vi "VSS Tangent.vi"(4 "Passe":bool, 6 "Cone de chute":dbl=0.55 format="%#_13g", 7 "IA State Input in":T1, 8 "distance between ball and robot":dbl=250.0 format="%#_13g", 9 "Ball":dbl[](array[numeric])=[-1986.6092529296875, -3009.6396484375], 10 "Target":dbl[](array[numeric]), 11 "R":dbl[](array[numeric])=[-2840.578369140625, -1536.7857666015625, -1.0371381044387817]) -> (1 "Destination":dbl[](array[numeric]))   [LabVIEW 2018]
uses:
  Core/AI Input.ctl
  Core/AI Robot.ctl
  Intel/Functions Enum.ctl
  Intel/AttackerStates.ctl
  Path Planning/RRT/PathDests.ctl
  Path Planning/RRT/PathDest.ctl
  Core/AI Ball.ctl
  Core/Field Size.ctl
  Core/AI Judge.ctl
  Intel/Command Enum.ctl
  Util/Events/Events.ctl
  <vilib>/Analysis/coordinate.llb/2D Cartesian Coordinate Rotation (Scalar).vi
  <vilib>/Analysis/NI_AALPro.lvlib
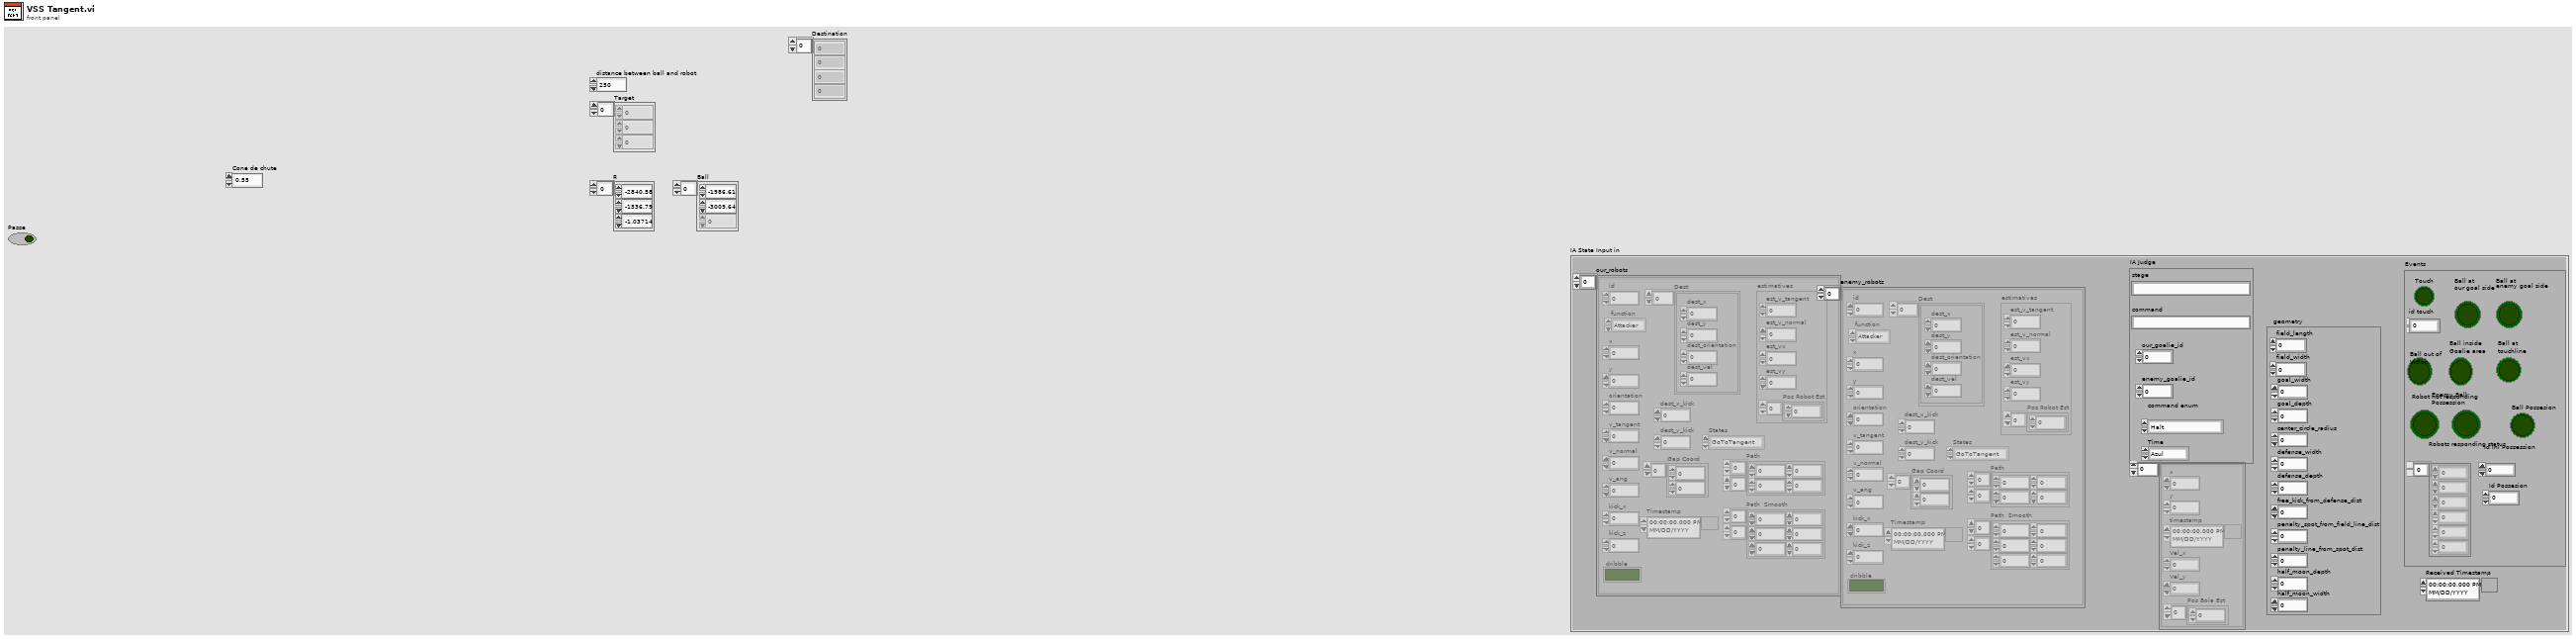
[diagram p1: front panel]
types:
  T1 = typedef "AI Input.ctl" = cluster{"our_robots":T2[], "enemy_robots":T2[], "balls":T7[], "geometry":T8, "IA Judge":T9, "Received Timestamp":timestamp, "Events":T11}
  T2 = typedef "AI Robot.ctl" = cluster{"id":u32, "function":T3, "x":dbl, "y":dbl, "orientation":dbl, "v_tangent":dbl, "v_normal":dbl, "v_ang":dbl, "kick_x":dbl, "kick_z":dbl, "dribble":bool, "Timestamp":timestamp, "estimatives":cluster{"est_v_tangent":dbl, "est_v_normal":dbl, "est_vx":dbl, "est_vy":dbl, "Pos Robot Est":dbl[]}, "dest_x_kick":dbl, "dest_y_kick":dbl, "Gap Coord":dbl[], "States":T4, "Path ":dbl[][], "Path  Smooth":dbl[][], "Dest":T5}
  T3 = typedef "Functions Enum.ctl" = enum16{"Attacker", "Goalie", "Defender", "Striker", "Goto 0", "Dummy", "Kicker", "ZigZag"}
  T4 = typedef "AttackerStates.ctl" = enum16{"Pass", "GoToTangent", "BallGetting", "GoToKick", "Rotate anti-clockwise", "Rotate Clockwise", ""}
  T5 = typedef "PathDests.ctl" = T6[]
  T6 = typedef "PathDest.ctl" = cluster{"dest_x":dbl, "dest_y":dbl, "dest_orientation":dbl, "dest_vel":dbl}
  T7 = typedef "AI Ball.ctl" = cluster{"x":dbl, "y":dbl, "timestamp":timestamp, "Vel_x":dbl, "Vel_y":dbl, "Pos Bola Est":dbl[]}
  T8 = typedef "Field Size.ctl" = cluster{"field_length":u32, "field_width":u32, "goal_width":u32, "goal_depth":u32, "center_circle_radius":u32, "defense_width":u32, "defense_depth":u32, "free_kick_from_defense_dist":u32, "penalty_spot_from_field_line_dist":u32, "penalty_line_from_spot_dist":u32, "half_moon_depth":u32, "half_moon_width":u32}
  T9 = typedef "AI Judge.ctl" = cluster{"stage":string, "command":string, "our_goalie_id":dbl, "enemy_goalie_id":dbl, "command enum":T10, "Time":enum16{"Azul", "Amarelo"}}
  T10 = typedef "Command Enum.ctl" = enum16{"Halt", "Stop", "Force Start", "PKA Normal Start", "Prepare Kickoff Ally", "PKE Normal Start", "Prepare Kickoff Enemy", "Prepare Penalty Ally", "PPA Normal Start", "Prepare Penalty Enemy", "PPE Normal Start", "Ball Placement Enemy Up", "Ball Placement Enemy Down", "Ball Placement Ally Up", "Ball Placement Ally Mid", "Ball Placement Ally Down", "Indirect Free Enemy", "Indirect Free Ally", "Timeout Enemy", "Timeout Ally", "Goal Enemy", "Goal Ally", "Normal Half Time", "Extra Time Break", "Extra Half Time", "None", "Post Game"}
  T11 = typedef "Events.ctl" = cluster{"Touch":bool, "id touch":dbl, "Ball out of \nVision":bool, "Ball inside \nGoalie area":bool, "Robot not responding":bool, "Robots responding status":dbl[], "Enemy Ball \nPossession":bool, "Id ini Possession":dbl, "Ball Possesion":bool, "Id Possesion":dbl, "Ball at\nour goal side":bool, "Ball at\ntouchline":bool, "Ball at\nenemy goal side":bool}
  T12 = enum16{"Frente", "Fundo", "Cima", "Baixo", "None"}
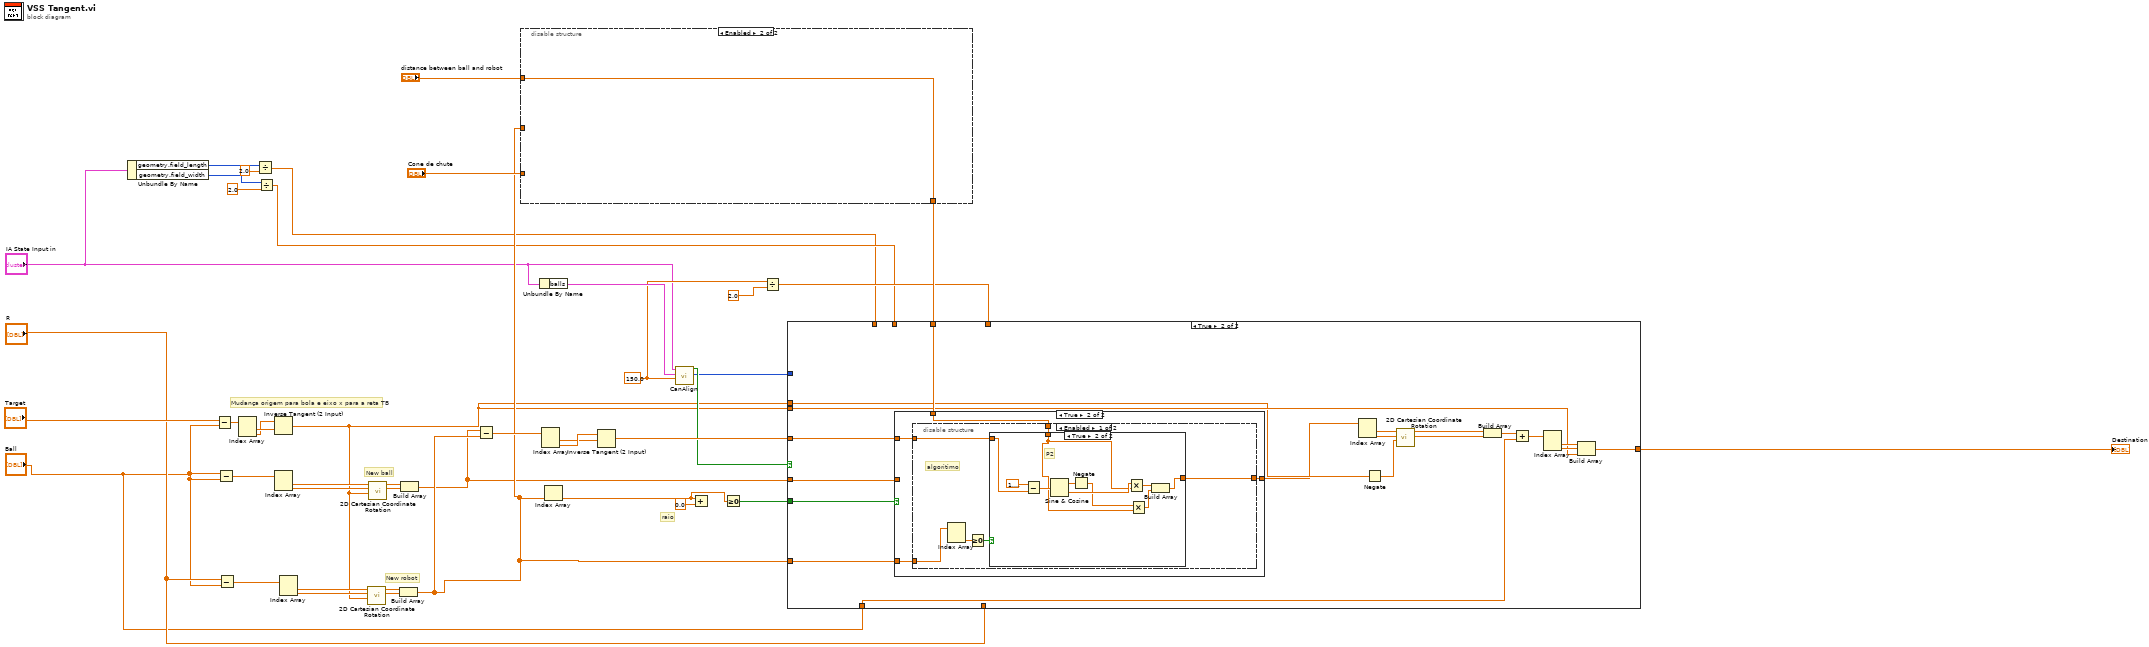
[diagram p0: block diagram]
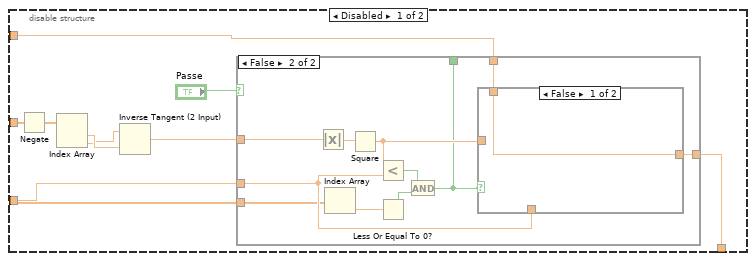
[diagram p2: hidden frame]
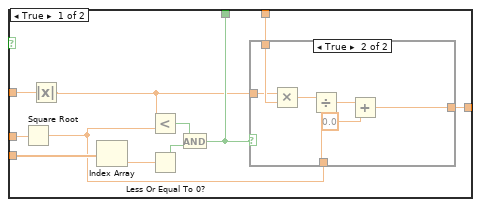
[diagram p3: hidden frame]
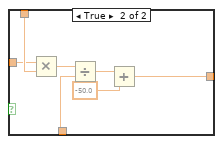
[diagram p5: hidden frame]
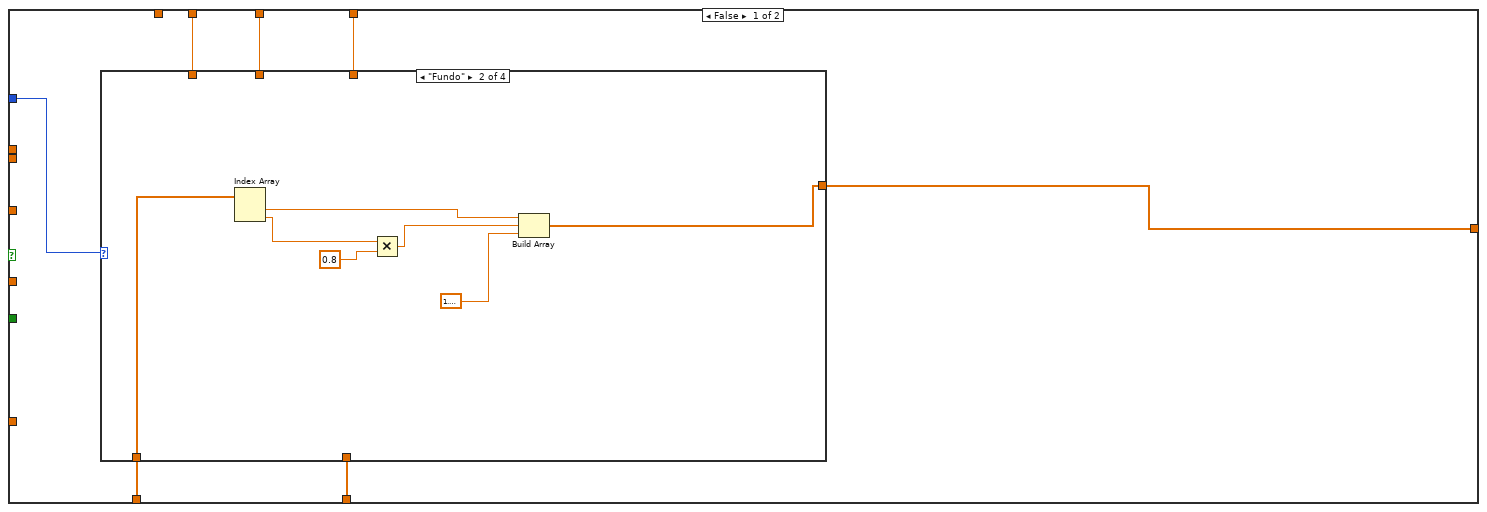
[diagram p6: hidden frame]
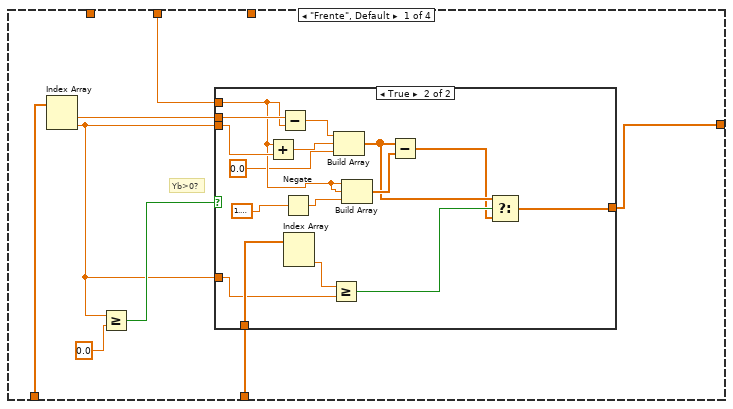
[diagram p7: hidden frame]
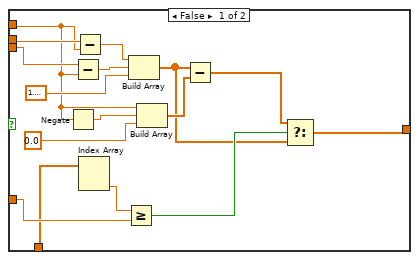
[diagram p8: hidden frame]
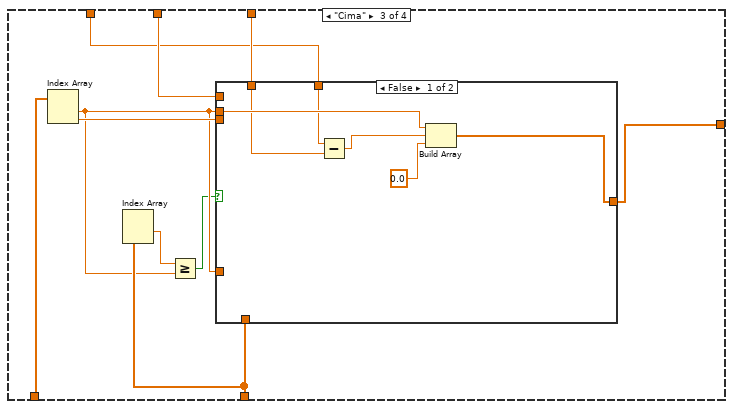
[diagram p9: hidden frame]
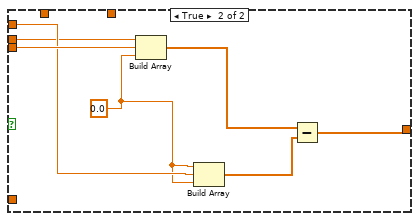
[diagram p10: hidden frame]
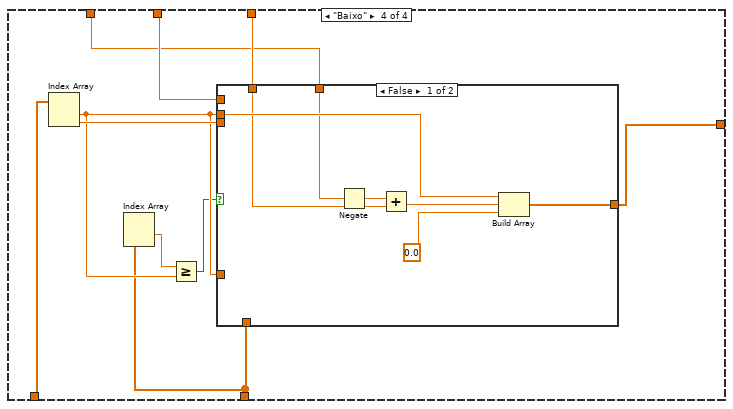
[diagram p11: hidden frame]
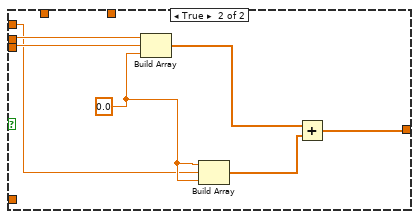
[diagram p12: hidden frame]
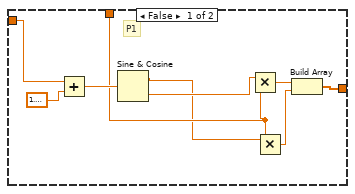
[diagram p14: hidden frame]
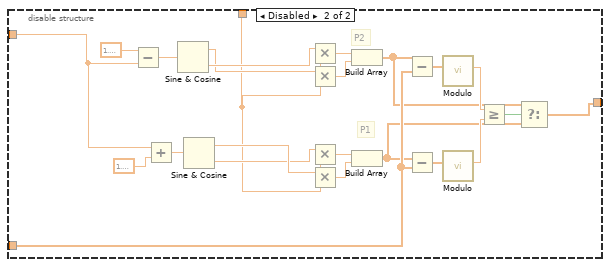
[diagram p15: hidden frame]
diagram:
  w12 = 150.0 ("Distância padrão\n de tolerância.")
  # "raio"
  # "New ball"
  # "New robot"
  # "Mudança origem para bola e eixo x para a reta TB"
  n1 = Unbundle By Name("IA State Input in") -> ("geometry.field_length"=w7:u32, "geometry.field_width"=w6:u32)
  n2 = Subtract(x="Target", y="Ball") -> (x-y=w37:dbl[])
  n3 = Subtract(x="Ball", y="Ball") -> (x-y=w41:dbl[])
  n4 = Subtract(x="R", y="Ball") -> (x-y=w38:dbl[])
  n5 = Index Array(array=w37) -> (element #1=w36:dbl, element #2=w35:dbl)  [unwired: 2 in]
  n6 = Divide(x=w7, y=2.0) -> (x/y=w4:dbl)
  n7 = Divide(x=w6, y=2.0) -> (x/y=w5:dbl)
  n8 = Inverse Tangent (2 Input)(1:w36, 2:w35) -> (0:w2:dbl)
  n9 = Index Array(array=w41) -> (element #1=w43:dbl, element #2=w42:dbl)  [unwired: 2 in]
  n10 = Index Array(array=w38) -> (element #1=w40:dbl, element #2=w39:dbl)  [unwired: 2 in]
  n11 = call-poly <vilib>:"2D Cartesian Coordinate Rotation.vi"("theta"=w2, "y"=w39, "x"=w40) -> ("y out"=w31:dbl, "x out"=w32:dbl)  [unwired: 6 in, 1 out]
  n12 = call-poly <vilib>:"2D Cartesian Coordinate Rotation.vi"("theta"=w2, "y"=w42, "x"=w43) -> ("y out"=w33:dbl, "x out"=w34:dbl)  [unwired: 6 in, 1 out]
  n13 = Build Array(w32, w31) -> (w23:dbl[])
  n14 = Build Array(w34, w33) -> (w15:dbl[])
  n15 = Subtract(x=w15, y=w23) -> (x-y=w28:dbl[])
  n16 = disable-structure shown="Enabled" {
    disable-tunnel: "Cone de chute" -> [w48 _]
    disable-tunnel: [w47 w91] -> w24
    disable-tunnel: w23 -> [w46 _]
    disable-tunnel: "distance between ball and robot" -> [w44 w91]
    frame Disabled {
      n17 = Negate(x=w46) -> (-x=w52:dbl[])
      n18 = Index Array(array=w52) -> (element #1=w51:dbl, element #2=w50:dbl)  [unwired: 2 in]
      n19 = Inverse Tangent (2 Input)(1:w51, 2:w50) -> (0:w49:dbl)
      n20 = case shown="False" "Passe" {
        tunnel: w49 -> [w63 w82]
        tunnel: w48 -> [w55 w81]
        tunnel: [w62 w80] -> w47
        tunnel: w44 -> [w61 w79]
        tunnel: w46 -> [w60 w76]
        tunnel: [w56 w72] -> _
        frame True {
          n21 = Square Root(x=w55) -> (sqrt(x)=w53:dbl)
          n22 = Absolute Value(x=w63) -> (abs(x)=w54:dbl)
          n23 = Index Array(array=w60) -> (element=w59:dbl)  [unwired: 1 in]
          n24 = Less?(x=w54, y=w53) -> (x < y?=w58:bool)
          n25 = Less Or Equal To 0?(x=w59) -> (x <= 0?=w57:bool)
          n26 = And(x=w58, y=w57) -> (x .and. y?=w56:bool)
          n27 = case shown="True" w56 {
            tunnel: w53 -> [_ w69]
            tunnel: [w64 w68] -> w62
            tunnel: w61 -> [w64 w67]
            tunnel: w54 -> [_ w66]
            frame False {
            }
            frame True {
              n28 = Multiply(x=w66, y=w67) -> (x*y=w71:dbl)
              n29 = Divide(x=w71, y=w69) -> (x/y=w70:dbl)
              n30 = Add(x=w70, y=0.0) -> (x+y=w68:dbl)
            }
          }
        }
        frame False {
          n31 = Absolute Value(x=w82) -> (abs(x)=w78:dbl)
          n32 = Index Array(array=w76) -> (element=w75:dbl)  [unwired: 1 in]
          n33 = Square(x=w78) -> (x^2=w77:dbl)
          n34 = Less?(x=w77, y=w81) -> (x < y?=w74:bool)
          n35 = Less Or Equal To 0?(x=w75) -> (x <= 0?=w73:bool)
          n36 = And(x=w74, y=w73) -> (x .and. y?=w72:bool)
          n37 = case shown="False" w72 {
            tunnel: w81 -> [_ w88]
            tunnel: [w83 w87] -> w80
            tunnel: w79 -> [w83 w86]
            tunnel: w77 -> [_ w85]
            frame False {
            }
            frame True {
              n38 = Multiply(x=w85, y=w86) -> (x*y=w90:dbl)
              n39 = Divide(x=w90, y=w88) -> (x/y=w89:dbl)
              n40 = Add(x=w89, y=-50.0) -> (x+y=w87:dbl)
            }
          }
        }
      }
    }
    frame Enabled {
    }
  }
  n41 = Unbundle By Name("IA State Input in") -> ("balls"=w18:T7[])
  n42 = Index Array(array=w28) -> (element #1=w29:dbl, element #2=w30:dbl)  [unwired: 2 in]
  n43 = Index Array(array=w23) -> (element=w20:dbl)  [unwired: 1 in]
  n44 = Inverse Tangent (2 Input)(1:w29, 2:w30) -> (0:w27:dbl)
  n45 = call "CanAlign.vi"("Distância padrão\n de tolerância."=w12, "balls"=w18, "IA State"="IA State Input in") -> ("Parede"=w16:T12, "CanAlign?"=w17:bool)  [unwired: 7 in]
  n46 = Add(x=w20, y=0.0) -> ()  [unwired: 1 out]
  n47 = Greater Or Equal To 0?(x=w20) -> (x >= 0?=w21:bool)
  n48 = Divide(x=w12, y=2.0) -> (x/y=w11:dbl)
  n49 = case shown="True" w17 {
    tunnel: [w92 w194] -> w1
    tunnel: w27 -> [_ w211]
    tunnel: w24 -> [w95 w210]
    tunnel: w23 -> [_ w209]
    tunnel: w21 -> [_ w208]
    tunnel: w16 -> [w98 _]
    tunnel: w15 -> [_ w207]
    tunnel: "Ball" -> [w97 w193]
    tunnel: "R" -> [w96 _]
    tunnel: w11 -> [w94 _]
    tunnel: w5 -> [w93 _]
    tunnel: w4 -> [_ _]
    tunnel: w2 -> [_ w197]
    tunnel: w2 -> [_ w196]
    frame False {
      n50 = case shown="\"Fundo\"" w98 {
        tunnel: w97 -> [w106 w145 w153 w171]
        tunnel: w96 -> [w103 _ w152 w170]
        tunnel: w95 -> [w100 _ w154 w173]
        tunnel: w94 -> [_ _ w150 w174]
        tunnel: w93 -> [_ _ w149 w172]
        tunnel: [w99 w139 w146 w169] -> w92
        frame "Frente", Default {
          # "Yb>0?"
          n51 = Index Array(array=w106) -> (element #1=w102:dbl, element #2=w101:dbl)  [unwired: 2 in]
          n52 = Greater Or Equal?(x=w101, y=0.0) -> (x >= y?=w104:bool)
          n53 = case shown="True" w104 {
            tunnel: w103 -> [w113 w138]
            tunnel: w101 -> [w116 w136]
            tunnel: w102 -> [w117 w134]
            tunnel: w101 -> [w110 w133]
            tunnel: w100 -> [w108 w130]
            tunnel: [w114 w125] -> w99
            frame False {
              n54 = Negate(x=w108) -> (-x=w109:dbl)
              n55 = Subtract(x=w110, y=w108) -> (x-y=w120:dbl)
              n56 = Subtract(x=w117, y=w108) -> (x-y=w121:dbl)
              n57 = Index Array(array=w113) -> (element #2=w115:dbl)  [unwired: 2 in, 1 out]
              n58 = Greater Or Equal?(x=w115, y=w116) -> (x >= y?=w122:bool)
              n59 = Build Array(w121, w120, 1.5707963267948966 ("element")) -> (w111:dbl[])
              n60 = Build Array(w108, w109, 0.0 ("element")) -> (w118:dbl[])
              n61 = Subtract(x=w111, y=w118) -> (x-y=w112:dbl[])
              n62 = Select(t=w112, s=w122, f=w111) -> (s? t:f=w114:dbl[])
            }
            frame True {
              n63 = Add(x=w130, y=w133) -> (x+y=w131:dbl)
              n64 = Subtract(x=w134, y=w130) -> (x-y=w132:dbl)
              n65 = Negate(x=1.5707963267948966 ("element")) -> (-x=w124:dbl)
              n66 = Index Array(array=w138) -> (element #2=w137:dbl)  [unwired: 2 in, 1 out]
              n67 = Greater Or Equal?(x=w137, y=w136) -> (x >= y?=w135:bool)
              n68 = Build Array(w132, w131, 0.0 ("element")) -> (w127:dbl[])
              n69 = Build Array(w130, w130, w124) -> (w128:dbl[])
              n70 = Subtract(x=w127, y=w128) -> (x-y=w126:dbl[])
              n71 = Select(t=w127, s=w135, f=w126) -> (s? t:f=w125:dbl[])
            }
          }
        }
        frame "Fundo" {
          n72 = Index Array(array=w145) -> (element #1=w143:dbl, element #2=w141:dbl)  [unwired: 2 in]
          n73 = Multiply(x=w141, y=0.8) -> (x*y=w142:dbl)
          n74 = Build Array(w143, w142, 1.5707963267948966 ("element")) -> (w139:dbl[])
        }
        frame "Cima" {
          n75 = Index Array(array=w153) -> (element #1=w151:dbl, element #2=w155:dbl)  [unwired: 2 in]
          n76 = Index Array(array=w152) -> (element #1=w148:dbl)  [unwired: 2 in, 1 out]
          n77 = Greater Or Equal?(x=w148, y=w151) -> (x >= y?=w147:bool)
          n78 = case shown="False" w147 {
            tunnel: w152 -> [_ _]
            tunnel: w151 -> [_ _]
            tunnel: w151 -> [w160 w162]
            tunnel: w155 -> [_ w166]
            tunnel: w154 -> [_ w164]
            tunnel: [w161 w165] -> w146
            tunnel: w150 -> [w158 _]
            tunnel: w149 -> [w157 _]
            frame False {
              n79 = Subtract(x=w157, y=w158) -> (x-y=w156:dbl)
              n80 = Build Array(w160, w156, 0.0 ("element")) -> (w161:dbl[])
            }
            frame True {
              w163 = 0.0 ("element")
              n81 = Build Array(w162, w166, w163) -> (w167:dbl[])
              n82 = Build Array(w163, w164, w163) -> (w168:dbl[])
              n83 = Subtract(x=w167, y=w168) -> (x-y=w165:dbl[])
            }
          }
        }
        frame "Baixo" {
          n84 = Index Array(array=w171) -> (element #1=w177:dbl, element #2=w178:dbl)  [unwired: 2 in]
          n85 = Index Array(array=w170) -> (element #1=w176:dbl)  [unwired: 2 in, 1 out]
          n86 = Greater Or Equal?(x=w176, y=w177) -> (x >= y?=w175:bool)
          n87 = case shown="False" w175 {
            tunnel: w170 -> [_ _]
            tunnel: w177 -> [_ _]
            tunnel: w177 -> [w184 w188]
            tunnel: w178 -> [_ w189]
            tunnel: w173 -> [_ w186]
            tunnel: [w185 w187] -> w169
            tunnel: w174 -> [w182 _]
            tunnel: w172 -> [w179 _]
            frame False {
              n88 = Negate(x=w179) -> (-x=w180:dbl)
              n89 = Add(x=w180, y=w182) -> (x+y=w181:dbl)
              n90 = Build Array(w184, w181, 0.0 ("element")) -> (w185:dbl[])
            }
            frame True {
              w190 = 0.0 ("element")
              n91 = Build Array(w188, w189, w190) -> (w191:dbl[])
              n92 = Build Array(w190, w186, w190) -> (w192:dbl[])
              n93 = Add(x=w191, y=w192) -> (x+y=w187:dbl[])
            }
          }
        }
      }
    }
    frame True {
      n94 = case shown="True" w208 {
        tunnel: w211 -> [_ w216]
        tunnel: [w212 w215] -> w195
        tunnel: w209 -> [_ w214]
        tunnel: w210 -> [_ w213]
        tunnel: w207 -> [w212 _]
        frame False {
        }
        frame True {
          n95 = disable-structure shown="Enabled" {
            disable-tunnel: w216 -> [w221 w252]
            disable-tunnel: [w220 w244] -> w215
            disable-tunnel: w214 -> [w218 w250]
            disable-tunnel: w213 -> [w217 w253]
            frame Enabled {
              # "algoritimo"
              n96 = Index Array(array=w218) -> (element #2=w222:dbl)  [unwired: 2 in, 1 out]
              n97 = Greater Or Equal To 0?(x=w222) -> (x >= 0?=w219:bool)
              n98 = case shown="True" w219 {
                tunnel: w221 -> [w226 w235]
                tunnel: [w228 w238] -> w220
                tunnel: w217 -> [w224 w234]
                frame False {
                  # "P1"
                  n99 = Add(x=w226, y=1.5707963267948966) -> (x+y=w227:dbl)
                  n100 = Sine & Cosine(0:w227) -> (1:w223:dbl, 2:w229:dbl)
                  n101 = Multiply(x=w229, y=w224) -> (x*y=w231:dbl)
                  n102 = Multiply(x=w223, y=w224) -> (x*y=w230:dbl)
                  n103 = Build Array(w231, w230) -> (w228:dbl[])
                }
                frame True {
                  # "P2"
                  n104 = Subtract(x=1.5707963267948966, y=w235) -> (x-y=w237:dbl)
                  n105 = Sine & Cosine(0:w237) -> (1:w233:dbl, 2:w241:dbl)
                  n106 = Negate(x=w233) -> (-x=w232:dbl)
                  n107 = Multiply(x=w241, y=w234) -> (x*y=w239:dbl)
                  n108 = Multiply(x=w232, y=w234) -> (x*y=w240:dbl)
                  n109 = Build Array(w239, w240) -> (w238:dbl[])
                }
              }
            }
            frame Disabled {
              # "P1"
              # "P2"
              n110 = Subtract(x=1.5707963267948966, y=w252) -> (x-y=w260:dbl)
              n111 = Add(x=w252, y=1.5707963267948966) -> (x+y=w255:dbl)
              n112 = Sine & Cosine(0:w260) -> (1:w263:dbl, 2:w264:dbl)
              n113 = Sine & Cosine(0:w255) -> (1:w257:dbl, 2:w256:dbl)
              n114 = Multiply(x=w264, y=w253) -> (x*y=w261:dbl)
              n115 = Multiply(x=w263, y=w253) -> (x*y=w262:dbl)
              n116 = Multiply(x=w256, y=w253) -> (x*y=w259:dbl)
              n117 = Multiply(x=w257, y=w253) -> (x*y=w258:dbl)
              n118 = Build Array(w261, w262) -> (w243:dbl[])
              n119 = Build Array(w259, w258) -> (w242:dbl[])
              n120 = Subtract(x=w243, y=w250) -> (x-y=w246:dbl[])
              n121 = Subtract(x=w242, y=w250) -> (x-y=w245:dbl[])
              n122 = call "Modulo.vi"("2D vector"=w246) -> ("Modulo"=w249:dbl)  [unwired: 10 in]
              n123 = call "Modulo.vi"("2D vector"=w245) -> ("Modulo"=w248:dbl)  [unwired: 10 in]
              n124 = Greater Or Equal?(x=w249, y=w248) -> (x >= y?=w247:bool)
              n125 = Select(t=w243, s=w247, f=w242) -> (s? t:f=w244:dbl[])
            }
          }
        }
      }
      n126 = Index Array(array=w195) -> (element #1=w198:dbl, element #2=w199:dbl)  [unwired: 2 in]
      n127 = Negate(x=w196) -> (-x=w206:dbl)
      n128 = call-poly <vilib>:"2D Cartesian Coordinate Rotation.vi"("theta"=w206, "y"=w199, "x"=w198) -> ("y out"=w201:dbl, "x out"=w200:dbl)  [unwired: 6 in, 1 out]
      n129 = Build Array(w200, w201) -> (w202:dbl[])
      n130 = Add(x=w202, y=w193) -> (x+y=w203:dbl[])
      n131 = Index Array(array=w203) -> (element #1=w204:dbl, element #2=w205:dbl)  [unwired: 2 in]
      n132 = Build Array(w204, w205, w197) -> (w194:dbl[])
    }
  }
  "Destination" <- w1
